vi "get_node_attribute_by_id.vi"(7 "node-id":refnum<class "ID.lvclass">, 8 "error in (no error)":errorcluster, 9 "default value (empty variant) in":variant, 10 "attribute-name":string, 11 "graph in":refnum<class "Graph.lvclass">) -> (0 "error out":errorcluster, 1 "default value (empty variant) out":variant, 2 "Boolean":bool, 3 "graph out":refnum<class "Graph.lvclass">)   [LabVIEW 2020, in "graph.lvlib" / "Graph.lvclass"]
uses:
  Graph.lvclass
  ID/ID.lvclass
  Graph.lvclass/Graph.ctl
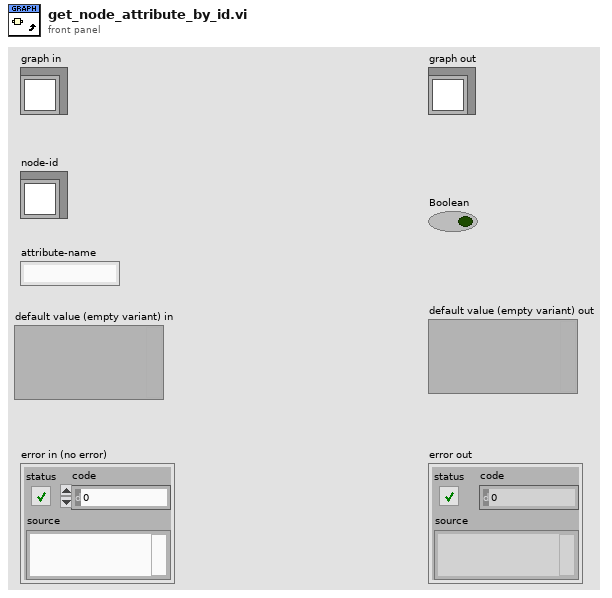
[diagram p1: front panel]
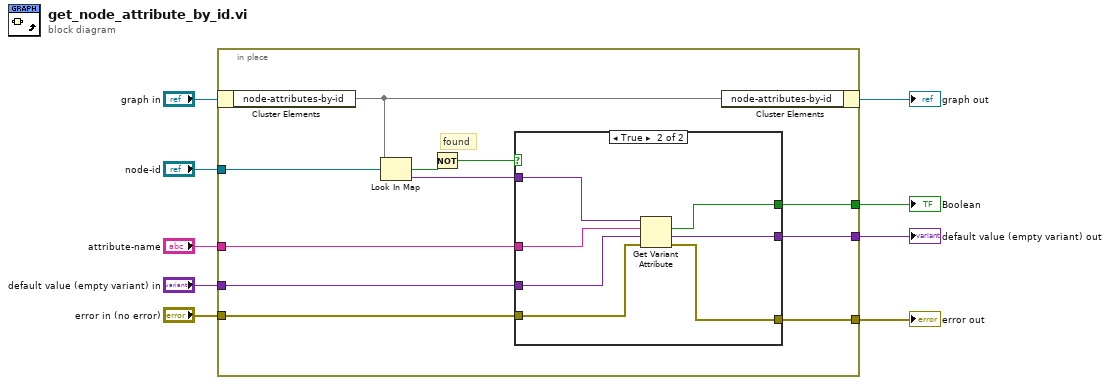
[diagram p0: block diagram]
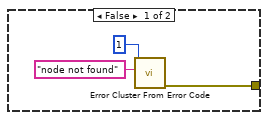
[diagram p2: hidden frame]
diagram:
  n1 = in-place {
    in-place-border: "attribute-name" -> [w17]
    in-place-border: "node-id" -> [w19]
    in-place-border: [w16] -> w3
    in-place-border: [w15] -> w4
    in-place-border: "default value (empty variant) in" -> [w14]
    in-place-border: [w12] -> w9
    in-place-border: "error in (no error)" -> [w11]
    # "found"
    n2 = in-place-cluster #1("graph in") -> ("node-attributes-by-id"=w20:map{refnum<class "ID.lvclass">, variant})
    n3 = Look In Map(map=w20, key=w19) -> (key not found?=w10:bool, value=w18:variant)  [unwired: 1 in]
    n4 = Not(x=w10) -> (.not. x?=w13:bool)
    n5 = case shown="True" w13 {
      tunnel: w18 -> [_ w30]
      tunnel: w17 -> [_ w29]
      tunnel: [_ w28] -> w16
      tunnel: [_ w27] -> w15
      tunnel: w14 -> [_ w26]
      tunnel: [w21 w25] -> w12
      tunnel: w11 -> [_ w24]
      frame False {
        n6 = call <vilib>:"Error Cluster From Error Code.vi"("error message (\"\")"="node not found" ("error message (\"\")"), "error code (0)"=1) -> ("error out"=w21:errorcluster)  [unwired: 7 in]
      }
      frame True {
        n7 = Get Variant Attribute(Variant=w30, name=w29, default value (empty Variant)=w26, error in=w24) -> (found=w27:bool, value=w28:variant, error out=w25:errorcluster)  [unwired: 1 out]
      }
    }
    n8 = in-place-cluster #1("node-attributes-by-id"=w20) -> (→"graph out":refnum<class "Graph.lvclass">)
  }
  "error out" <- w9
  "Boolean" <- w4
  "default value (empty variant) out" <- w3
